vi "Drive Controller.vi"(8 "error in":errorcluster) -> ()   [LabVIEW 2020]
doc: "This VI executes continuously carrying out the current operation and responding to updates or new operation requests. It will often contain the timing or control code that is difficult to place directly in TeleOp. This VI generally opens all sensors and motors and isolates the rest of the robot code from knowing implementation details of how the operations are carried out."
uses:
  <vilib>/Rock Robotics/WPI/Framework/Completion Status.ctl
  Drive Setpoints.ctl
  Drive Operations.ctl
  <vilib>/Rock Robotics/WPI/SafetyOutput/WPI_SafetyOutputConfigMenu.ctl
  <vilib>/Rock Robotics/WPI/RobotDrive/WPI_RobotDriveOpen2MotorWithExistingMotors.vi
panel:
  in  "Interactive Values":T1
  in  "Buttons":cluster{"Execute Cmd":bool, "Abort Cmd":bool}
  out "Command Timing":cluster{"Start Time (ms)":u32, "Iterations":i32}
  out "Status":T3
  out "Setpoints":T4(graph)
  out "Current\nCmd":string
  # "Tip: The graph shows the motor setpoints. It may also be helpful to observe inputs and sensor values.\nYou may also want to display tuning or debugging controls."
  # "Interactive Command: You may fill in the settings for a command\nand schedule it with the Execute button. You can observe and abort\nany command while fine tuning the code for the controller."
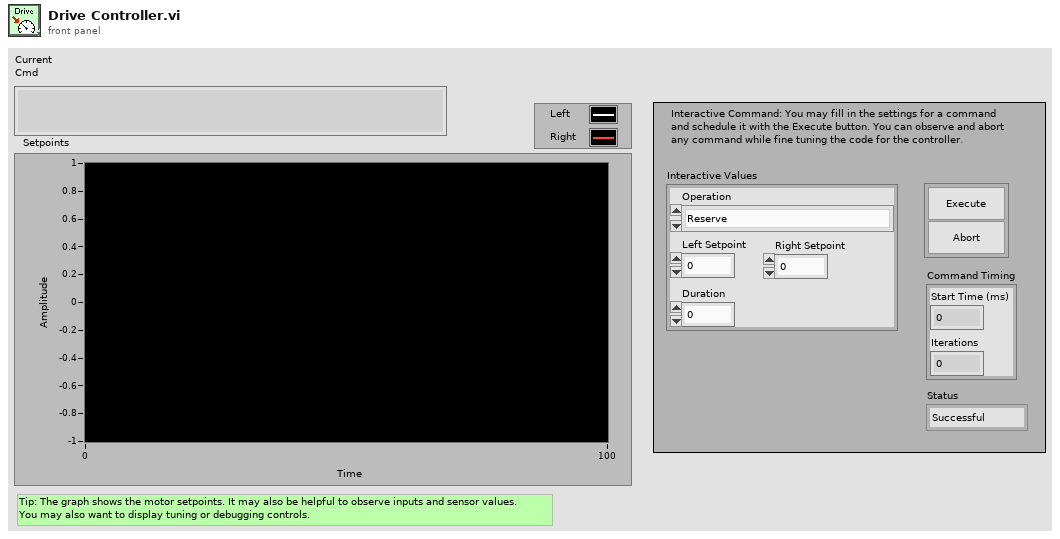
[diagram p1: front panel]
types:
  T1 = typedef "Drive Setpoints.ctl" = cluster{"Operation":T2, "Left Setpoint":dbl, "Right Setpoint":dbl, "Duration":dbl}
  T2 = typedef "Drive Operations.ctl" = enum16{"Reserve", "Read Current", "Immediate", "Drive for Time", "Drive for Distance"}
  T3 = typedef "Completion Status.ctl" = enum16{"Successful", "Aborted", "Incomplete"}
  T4 = cluster{"Left Setpoint":dbl, "Right Setpoint":dbl}
  T5 = typedef "WPI_SafetyOutputConfigMenu.ctl" = enum16{"Enable", "Disable"}
  T6 = typedef "WPI_MotorControlDeviceRef.ctl" = cluster{"DeviceStatus":errorcluster, "Type":T7, "PWM":cluster{"PWM Channel":T8, "DeadBand":T9}, "CAN":cluster{"Device Number":u8, "SetOutput VI Ref":variant, "GetOutput VI Ref":variant, "Enable VI Ref":variant, "Disable VI Ref":variant, "Data":variant}, "Invert":bool, "DIO PWM":cluster{"PWM \"Enable\" Channel":T8, "DIOChannel":T10, "PWM Rate":dbl}}
  T7 = typedef "WPI_MotorControlType.ctl" = enum16{"PWM", "CAN", "DIO PWM"}
  T8 = typedef "FPGA_DIOPWMChannel.ctl" = enum8{"PWM 0", "PWM 1", "PWM 2", "PWM 3", "PWM 4", "PWM 5", "PWM 6", "PWM 7", "PWM 8", "PWM 9", "PWM MXP 0", "PWM MXP 1", "PWM MXP 2", "PWM MXP 3", "PWM MXP 4", "PWM MXP 5", "PWM MXP 6", "PWM MXP 7", "PWM MXP 8", "PWM MXP 9", "Invalid"}
  T9 = typedef "WPI_PWMDeadband.ctl" = cluster{"Name":string, "maxPositivePwm":i32, "minPositivePwm":i32, "centerPwm":i32, "maxNegativePwm":i32, "minNegativePwm":i32, "angularRange":u16}
  T10 = typedef "FPGA_DIOChannel.ctl" = enum8{"DIO 0", "DIO 1", "DIO 2", "DIO 3", "DIO 4", "DIO 5", "DIO 6", "DIO 7", "DIO 8", "DIO 9", "DIO MXP 0", "DIO MXP 1", "DIO MXP 2", "DIO MXP 3", "DIO MXP 4", "DIO MXP 5", "DIO MXP 6", "DIO MXP 7", "DIO MXP 8", "DIO MXP 9", "DIO MXP 10", "DIO MXP 11", "DIO MXP 12", "DIO MXP 13", "DIO MXP 14", "DIO MXP 15", "SPI Port CS1", "SPI Port CS2", "SPI Port CS3", "SPI Port MISO", "SPI Port MOSI", "Invalid"}
  T11 = typedef "WPI_RobotDriveDevRef.ctl" = cluster{"DevStatus":errorcluster, "Motors[]":T6[], "Square Inputs":bool, "Max Output":dbl}
  T12 = typedef "Command Status Info.ctl" = cluster{"Name":string, "Status":T3, "notifier out":T13}
  T13 = typedef "Completion Notifier.ctl" = refnum<notifier>
  T14 = cluster{"SubSystem Data":T1, cluster{"Start Time (ms)":u32, "Iterations":i32}, cluster{"Command Info":T12, "Description":string, "Default Command":T1, "queue out":refnum<queue>, "Subsystem Name":string}}
  T15 = cluster{"SubSystem Data":T1, cluster{"Start Time (ms)":u32, "Iterations":i32}, "Default Command Arguments":cluster{"Command Info":T12, "Description":string, "Default Command":T1, "queue out":refnum<queue>, "Subsystem Name":string}}
  T16 = cluster{"Don't move motors while reserved":dbl, "Don't move motors while reserved":dbl}
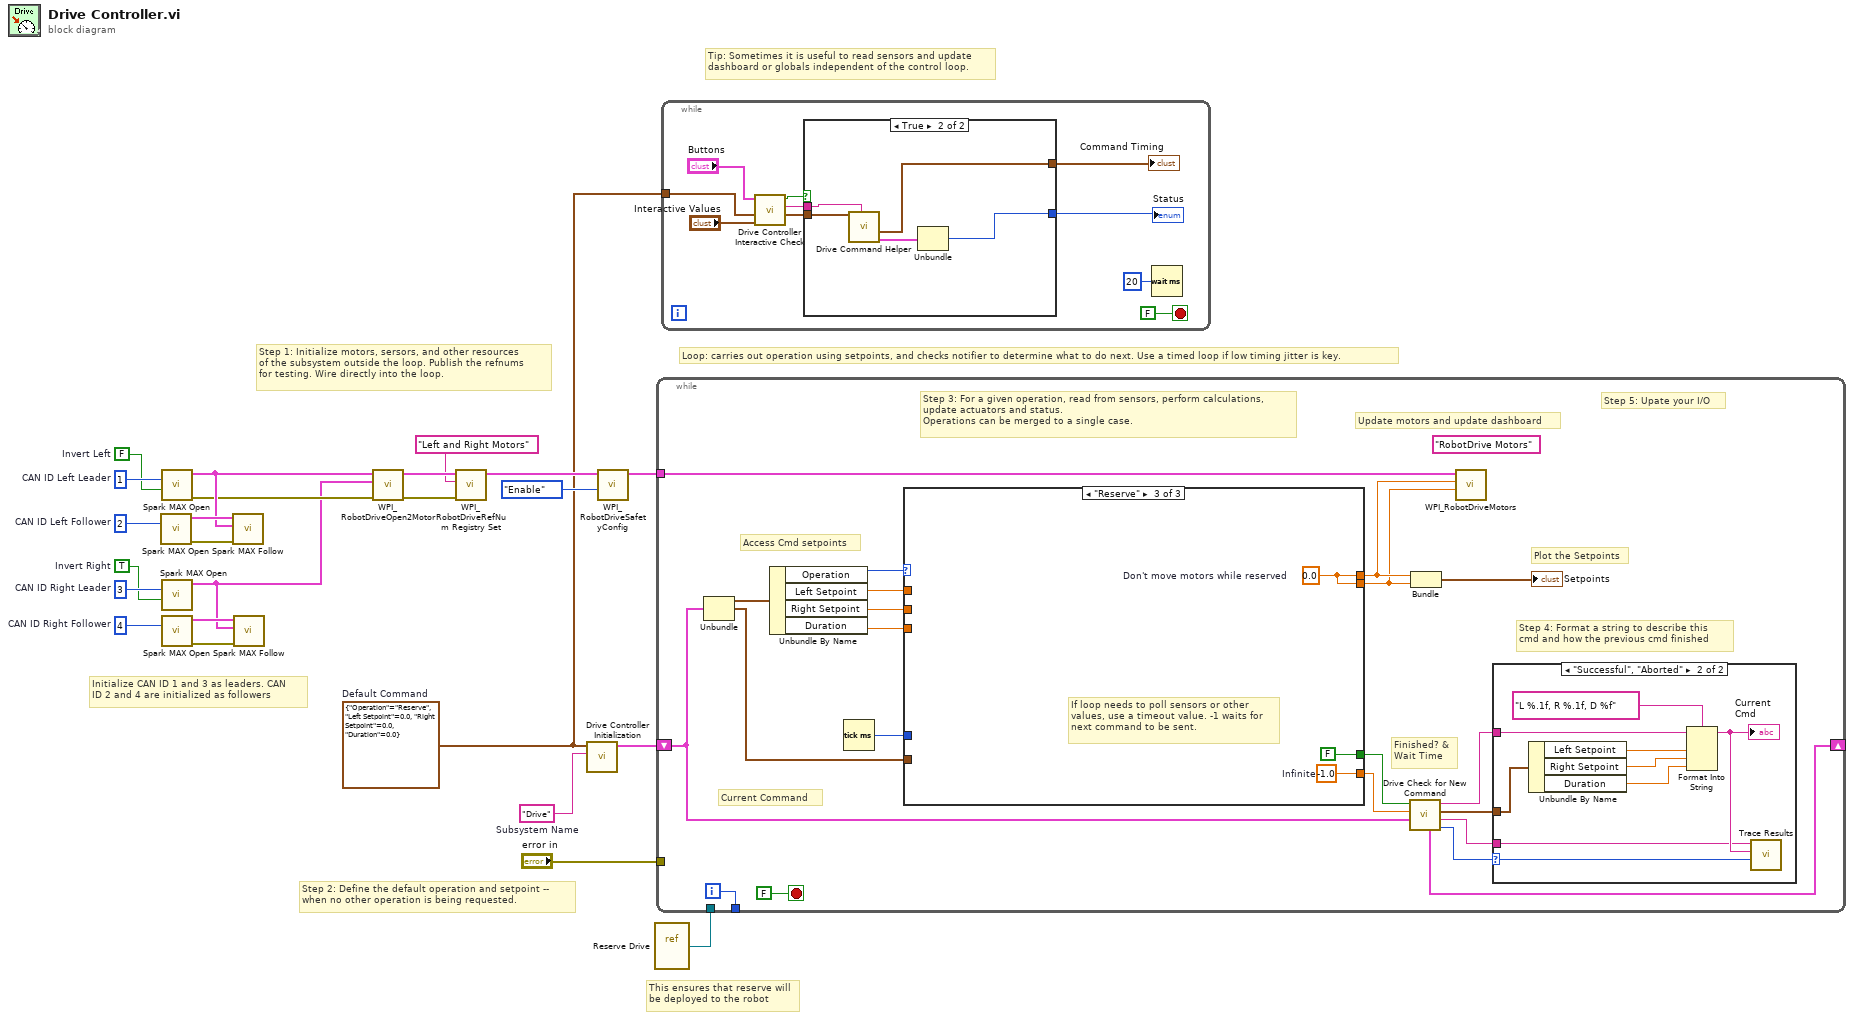
[diagram p0: block diagram]
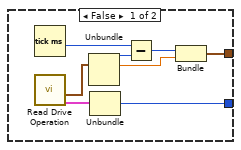
[diagram p2: hidden frame]
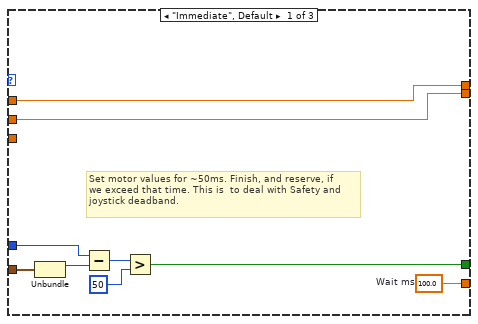
[diagram p4: hidden frame]
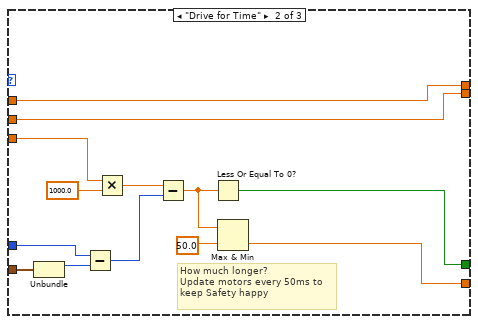
[diagram p5: hidden frame]
diagram:
  w4 = FALSE  # Invert Left
  w5 = TRUE  # Invert Right
  w7 = u8 3  # CAN ID Right Leader
  w6 = u8 4  # CAN ID Right Follower
  w12 = u8 1  # CAN ID Left Leader
  w13 = u8 2  # CAN ID Left Follower
  w14 = T1 {"Operation"=enum."Reserve", "Left Setpoint"=0.0, "Right Setpoint"=0.0, "Duration"=0.0}  # Default Command
  w24 = "Drive"  # Subsystem Name
  # "Initialize CAN ID 1 and 3 as leaders. CAN \nID 2 and 4 are initialized as followers"
  # "This ensures that reserve will\nbe deployed to the robot"
  # "Tip: Sometimes it is useful to read sensors and update\ndashboard or globals independent of the control loop."
  # "Step 2: Define the default operation and setpoint --\nwhen no other operation is being requested."
  # "Step 1: Initialize motors, sersors, and other resources\nof the subsystem outside the loop. Publish the refnums\nfor testing. Wire directly into the loop."
  # "Loop: carries out operation using setpoints, and checks notifier to determine what to do next. Use a timed loop if low timing jitter is key."
  n1 = call <vilib>:"Spark MAX Open.vi"("Device Number"=w13) -> ("error out"=w10:errorcluster, "MotorControlDeviceRef"=w11:T6)  [unwired: 9 in]
  n2 = call <vilib>:"Spark MAX Open.vi"("Invert"=w4, "Device Number"=w12) -> ("error out"=w2:errorcluster, "MotorControlDeviceRef"=w3:T6)  [unwired: 8 in]
  n3 = call <vilib>:"Spark MAX Open.vi"("Invert"=w5, "Device Number"=w7) -> ("MotorControlDeviceRef"=w1:T6)  [unwired: 8 in, 1 out]
  n4 = call <vilib>:"Spark MAX Open.vi"("Device Number"=w6) -> ("error out"=w9:errorcluster, "MotorControlDeviceRef"=w8:T6)  [unwired: 9 in]
  n5 = call <vilib>:"Spark MAX Follow.vi"("error in (no error)"=w10, "Master Controller"=w3, "MotorControlDeviceRef"=w11) -> ()  [unwired: 7 in, 2 out]
  n6 = call <vilib>:"Spark MAX Follow.vi"("error in (no error)"=w9, "Master Controller"=w1, "MotorControlDeviceRef"=w8) -> ()  [unwired: 7 in, 2 out]
  n7 = call-poly <vilib>:"WPI_RobotDriveOpen2Motor.vi"("error in (no error)"=w2, "Right Motor Dev Ref"=w1, "Left Motor Dev Ref"=w3) -> ("error out"=w21:errorcluster, "RobotDriveDevRef"=w23:T11)  [unwired: 2 in, 5 out]
  n8 = call <vilib>:"WPI_RobotDriveRefNum Registry Set.vi"("error in (no error)"=w21, "refnum name"="Left and Right Motors", "RobotDriveDevRef"=w23) -> ("RobotDriveDevRef"=w20:T11)  [unwired: 1 in, 7 out]
  n9 = call "Drive Controller Initialization.vi"("Subsystem Name"=w24, "Default Command"=w14) -> ("Current Command"=w16:T14)  [unwired: 9 in]
  n10 = call <vilib>:"WPI_RobotDriveSafetyConfig.vi"("mode"=WPI_SafetyOutputConfigMenu."Enable", "RobotDriveDevRef"=w20) -> ("RobotDriveDevRef"=w18:T11)  [unwired: 8 in, 1 out]
  n11 = vi-ref "Reserve Drive.vi"() -> (w15:refnum<vi>)
  n12 = while {
    shift-right: [w32] -> _
    shift-left: w16 -> [w25]
    tunnel: [w44] -> _
    tunnel: w18 -> [w40]
    tunnel: "error in" -> [_]
    tunnel: w15 -> [_]
    i -> [w44]
    stop <- FALSE stop-if-true
    (unwired) "RobotDrive Motors" ("Name")
    # "Step 5: Upate your I/O"
    # "Step 4: Format a string to describe this\ncmd and how the previous cmd finished"
    # "Current Command"
    # "Update motors and update dashboard"
    # "Plot the Setpoints"
    # "Access Cmd setpoints"
    # "Finished? &\nWait Time"
    # "Step 3: For a given operation, read from sensors, perform calculations,\nupdate actuators and status.\nOperations can be merged to a single case."
    n13 = Unbundle(w25) -> ("SubSystem Data"=w39:T1, w26:cluster{"Start Time (ms)":u32, "Iterations":i32})  [unwired: 1 out]
    n14 = Unbundle By Name(w39) -> ("Operation"=w38:T2, "Left Setpoint"=w37:dbl, "Right Setpoint"=w36:dbl, "Duration"=w35:dbl)
    n15 = Tick Count (ms)() -> (millisecond timer value=w34:u32)
    n16 = case shown="\"Reserve\"" w38 {
      tunnel: [w63 w64 w79] -> w31
      tunnel: [w56 w71 FALSE ("ignore previous (F)")] -> w30
      tunnel: w26 -> [w55 w73 _]
      tunnel: [w62 w70 w77] -> w42
      tunnel: [w61 w69 w77] -> w41
      tunnel: w37 -> [w62 w70 _]
      tunnel: w36 -> [w61 w69 _]
      tunnel: w35 -> [_ w68 _]
      tunnel: w34 -> [w57 w67 _]
      frame "Immediate", Default {
        w63 = 100.0  # Wait ms
        # "Set motor values for ~50ms. Finish, and reserve, if\nwe exceed that time. This is  to deal with Safety and\njoystick deadband."
        n17 = Unbundle(w55) -> ("Start Time (ms)"=w58:u32)  [unwired: 1 out]
        n18 = Subtract(x=w57, y=w58) -> (x-y=w59:u32)
        n19 = Greater?(x=w59, y=u8 50 ("Left Motor")) -> (0:w56:bool)
      }
      frame "Drive for Time" {
        # "How much longer?\nUpdate motors every 50ms to\nkeep Safety happy"
        n20 = Unbundle(w73) -> ("Start Time (ms)"=w72:u32)  [unwired: 1 out]
        n21 = Subtract(x=w67, y=w72) -> (x-y=w76:u32)
        n22 = Multiply(x=w68, y=1000.0) -> (x*y=w75:dbl)
        n23 = Subtract(x=w75, y=w76) -> (x-y=w66:dbl)
        n24 = Less Or Equal To 0?(x=w66) -> (x <= 0?=w71:bool)
        n25 = Max & Min(x=w66, y=50.0) -> (min(x,y)=w64:dbl)  [unwired: 1 out]
      }
      frame "Reserve" {
        w77 = 0.0  # Don't move motors while reserved
        w79 = -1.0  # Infinite
        # "If loop needs to poll sensors or other\nvalues, use a timeout value. -1 waits for\nnext command to be sent."
      }
    }
    n26 = call "Drive Check for New Command.vi"("input cluster"=w25, "Wait time (ms)"=w31, "Finished?"=w30) -> ("Completion"=w33:T3, "Subsystem Name"=w27:string, "Current Command"=w28:T1, "Initial Trace String"=w29:string, "Next Command"=w32:T15)  [unwired: 4 in]
    n27 = Bundle("Don't move motors while reserved"=w42, "Don't move motors while reserved"=w41) -> (→"Setpoints":T16)  [unwired: 1 in]
    n28 = call <vilib>:"WPI_RobotDriveMotors.vi"("RightSpeed"=w41, "LeftSpeed"=w42, "RobotDriveDevRef"=w40) -> ()  [unwired: 1 in, 8 out]
    n29 = case shown="\"Successful\", \"Aborted\"" w33 {
      selector: w33 -> [_ w54]
      tunnel: w29 -> [_ w49]
      tunnel: w28 -> [_ w50]
      tunnel: w27 -> [_ w46]
      frame "Incomplete", Default {
        # "Continuing current command"
      }
      frame "Successful", "Aborted" {
        # "Report and setup for next command"
        n30 = Unbundle By Name(w50) -> ("Left Setpoint"=w52:dbl, "Right Setpoint"=w53:dbl, "Duration"=w47:dbl)
        n31 = Format Into String(format string="L %.1f, R %.1f, D %f", initial string=w49, w52, w53, w47) -> (resulting string=w48:string)  [unwired: 1 in, 1 out]
        "Current\nCmd" <- w48
        n32 = call <vilib>:"Trace Results.vi"("Status of previous command"=w54, "Description"=w48, "Subsystem"=w46) -> ()  [unwired: 9 in]
      }
    }
  }
  n33 = while {
    tunnel: w14 -> [w81]
    stop <- FALSE stop-if-true
    n34 = call "Drive Controller Interactive Check.vi"("Interactive Command In"="Interactive Values", "Default Command"=w81, "Buttons"="Buttons") -> ("Interactive Command Out"=w83:T1, "Trace String"=w84:string, "Schedule"=w85:bool)  [unwired: 6 in]
    n35 = case shown="True" w85 {
      tunnel: [w94 w102] -> w86
      tunnel: [w93 w98] -> w87
      tunnel: w84 -> [_ w100]
      tunnel: w83 -> [_ w99]
      frame False {
        n36 = Tick Count (ms)() -> (millisecond timer value=w97:u32)
        n37 = call "Read Drive Operation.vi"() -> ("Command Info"=w91:T12, "SubSystem Data"=w90:T1)  [unwired: 9 in, 1 out]
        n38 = Unbundle(w90) -> ("Operation"=w95:T2, "Left Setpoint"=w92:dbl)  [unwired: 2 out]
        n39 = Unbundle(w91) -> ("Status"=w94:T3)  [unwired: 2 out]
        n40 = Subtract(x=w97, y=w95) -> (x-y=w96:u32)
        n41 = Bundle(w96, "Left Setpoint"=w92) -> (w93:cluster{u32, "Left Setpoint":dbl})  [unwired: 1 in]
      }
      frame True {
        n42 = call "Drive Command Helper.vi"("Description"=w100, "SubSystem Data"=w99) -> ("Command Info Out"=w101:T12, "Command Timing"=w98:cluster{"Start Time (ms)":u32, "Iterations":i32})  [unwired: 7 in, 1 out]
        n43 = Unbundle(w101) -> ("Status"=w102:T3)  [unwired: 2 out]
      }
    }
    "Status" <- w86
    "Command Timing" <- w87
    n44 = Wait (ms)(milliseconds to wait=u32 20) -> ()  [unwired: 1 out]
  }
